vi "Hardware-Knock-Host.vi"() -> ()   [LabVIEW 2016]
panel:
  in  "_Hidden":enum32{"Page 1"}(tab)
  in  "CylinderOffsets":sgl[](array[numeric])=[0.0, 0.0, 0.0, 0.0, 0.0, 0.0, 0.0, 0.0, 0.0, 0.0, 0.0, 0.0, 0.0, 0.0, 0.0, 0.0]
  in  "SensorSelect":i32[](array[numeric])=[0, 0, 0, 0, 0, 0, 0, 0, 0, 0, 0, 0, 0, 0, 0, 0]
  out "Knock":u32
  out "KnockIntensity":sgl[](array[numeric])
  in  "_Refresh":bool
  in  "_Knock Channels":i32(listbox) caption="Summary"
  in  "_Cylinder Offset":sgl caption="Cylinder Offset"
  in  "_Knock Sensor Select":i32(ring) caption="Sensor Select" items=["None"=-1, "Sensor 1"=0, "Sensor 2"=1, "Sensor 3"=2, "Sensor 4"=3, "Sensor 5"=4, "Sensor 6"=5, "Sensor 7"=6, "Sensor 8"=7, "Sensor 9"=8, "Sensor 10"=9, "Sensor 11"=10, "Sensor 12"=11]
  in  "Threshold":sgl=2.0 caption="[]"
  in  "HighCutoff":sgl=6000.0 caption="[]" format="%#_6p"
  in  "LowCutoff":sgl=5000.0 caption="[]" format="%#_6p"
  in  "RefStart":sgl=-70.0 caption="[]"
  in  "RefEnd":sgl=-90.0 caption="[]"
  in  "KnockEnd":sgl=20.0 caption="[DBTDC]"
  in  "KnockStart":sgl caption="[]"
  # "Knock Settings"
  # "[CAD]"
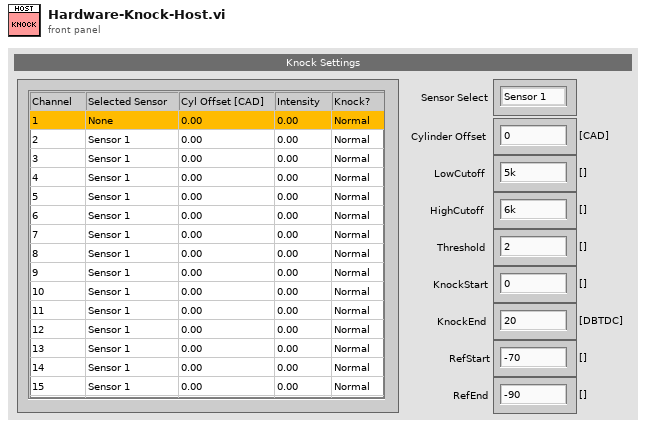
[diagram p1: front panel]
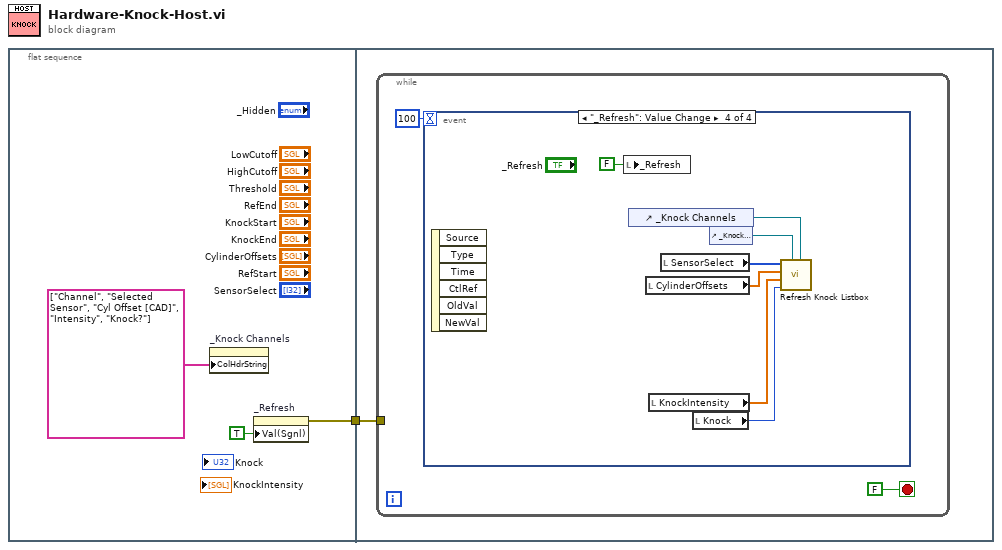
[diagram p0: block diagram]
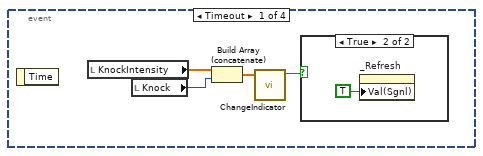
[diagram p2: hidden frame]
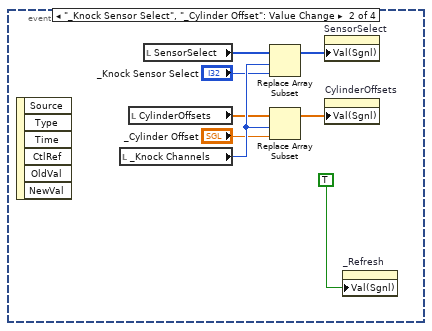
[diagram p4: hidden frame]
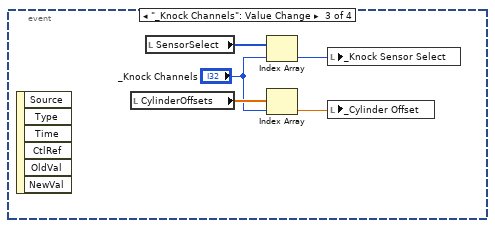
[diagram p5: hidden frame]
diagram:
  n1 = flat-sequence {
    tunnel: [w2] -> w1
    tunnel: w1 -> [w5]
    frame #0 {
      n2 = property on="_Knock Channels" class="MCListbox (strict)"("ColHdrString"=string[] ["Channel", "Selected Sensor", "Cyl Offset [CAD]", "Intensity", "Knock?"] ("Column Header Strings[] 2")) -> ()  [unwired: 2 in, 2 out]
      n3 = property on="_Refresh" class="Bool (strict)"("Val(Sgnl)"=TRUE ("Value (Signaling)")) -> (error out=w2:errorcluster)  [unwired: 2 in, 1 out]
    }
    frame #1 {
      n4 = while {
        tunnel: w5 -> [_]
        stop <- FALSE stop-if-true
        n5 = event shown="[3] \"_Refresh\": Value Change" {
          selector: _ -> [_ _ _ _]
          dyn-events: _ -> [_ _ _ _]
          timeout: 100 -> [_ _ _ _]
          event Timeout {
            n6 = event-data() -> ()  [unwired: 1 in, 1 out]
            n7 = local read "KnockIntensity"() -> (w8:sgl[])
            n8 = local read "Knock"() -> (w9:u32)
            n9 = Build Array (concatenate)(w8, w9) -> (w10:sgl[])
            n10 = call "ChangeIndicator.vi"("Input"=w10) -> ("Change"=w11:bool)  [unwired: 9 in]
            n11 = case shown="True" w11 {
              frame False {
              }
              frame True {
                n12 = property on="_Refresh" class="Bool (strict)"("Val(Sgnl)"=TRUE ("Value (Signaling)")) -> ()  [unwired: 2 in, 2 out]
              }
            }
          }
          event "_Knock Sensor Select", "_Cylinder Offset": Value Change {
            n13 = event-data() -> ()  [unwired: 1 in, 6 out]
            n14 = local read "_Knock Channels"() -> (w18:i32)
            n15 = local read "CylinderOffsets"() -> (w17:sgl[])
            n16 = local read "SensorSelect"() -> (w20:i32[])
            n17 = Replace Array Subset(array=w20, new element="_Knock Sensor Select", index=w18) -> (w19:i32[])
            n18 = Replace Array Subset(array=w17, new element="_Cylinder Offset", index=w18) -> (w16:sgl[])
            n19 = property on="SensorSelect" class="Arr (strict)"("Val(Sgnl)"=w19) -> ()  [unwired: 2 in, 2 out]
            n20 = property on="CylinderOffsets" class="Arr (strict)"("Val(Sgnl)"=w16) -> ()  [unwired: 2 in, 2 out]
            n21 = property on="_Refresh" class="Bool (strict)"("Val(Sgnl)"=TRUE ("Value (Signaling)")) -> ()  [unwired: 2 in, 2 out]
          }
          event "_Knock Channels": Value Change {
            n22 = event-data() -> ()  [unwired: 1 in, 6 out]
            n23 = local read "CylinderOffsets"() -> (w24:sgl[])
            n24 = local read "SensorSelect"() -> (w25:i32[])
            n25 = Index Array(array=w25, index="_Knock Channels") -> (element=w22:i32)
            n26 = Index Array(array=w24, index="_Knock Channels") -> (element=w21:sgl)
            n27 = local write "_Knock Sensor Select"(w22) -> ()
            n28 = local write "_Cylinder Offset"(w21) -> ()
          }
          event "_Refresh": Value Change {
            n29 = event-data() -> ()  [unwired: 1 in, 6 out]
            n30 = local write "_Refresh"(FALSE ("_Refresh")) -> ()
            n31 = control-ref of="_Knock Channels"() -> (w26:refnum<vi>)
            n32 = local read "CylinderOffsets"() -> (w29:sgl[])
            n33 = local read "KnockIntensity"() -> (w30:sgl[])
            n34 = local read "SensorSelect"() -> (w28:i32[])
            n35 = local read "Knock"() -> (w31:u32)
            n36 = control-ref of="_Knock Sensor Select"() -> (w27:refnum<vi>)
            n37 = call "Refresh Knock Listbox.vi"("Knock Listbox Refnum"=w26, "Knock Sensor Refnum"=w27, "Knock"=w31, "KnockIntensity"=w30, "CylinderOffsets"=w29, "SensorSelect"=w28) -> ()  [unwired: 6 in]
          }
        }
      }
    }
  }
